vi "ATS_State_Device.vi"(6 "DevInfo_In":T3={"Handle"=0, "Board"="", "CPLD"="", "MemorySize"=0, "SampleSize"=0, "ID"=0, "High_Memory"=FALSE, "Chan/Board"=2}, 7 "Sys_In":T1={"MS_Mode"=FALSE, "MBoard"=0, "#Board"=1}, 8 "Ref_In":T2 {"Ranges (v)" format="%.2e"; "RangeB (v)" format="%.2e"; "RangeA (v)" format="%.2e"; "Clock (s)" format="%.2e"}, 9 "SetupIn":T5={"Record"={"Count"=1, "Presize"=512, "Length"=4096}, "Clock"={"ClckSource"=enum."Internal", "ClckRate"=16, "ClckEdge"=0, "Decimation"=0}, "Inputs"=[], "Trigger"={"TrigOperation"=enum."Only X", "Timeout (s)"=1.0, "Trig. Delay"=0, "Engine X"={"Source"=enum."Chan_A", "Slope"=enum."Positive", "Level"=128}, "Engine Y"={"Source"=enum."Disable", "Slope"=enum."Positive", "Level"=128}, "ExtTrigControl"={"Coupling"=enum."AC", "Range"=enum."1 V"}}} {"Inputs"."Range" items=["20mV", "40mV", "50mV", "80mV", "100mV", "200mV", "400mV", "500mV", "800mV", "1 V", "1.25 V", "2 V", "4 V", "5 V", "8 V", "10 V", "16 V", "20 V", "40 V", "HiFi"]; "Clock"."ClckEdge" items=["Rising", "Falling"]; "Clock"."ClckRate" items=["1 kS/s", "2 kS/s", "5 kS/s", "10 kS/s", "20 kS/s", "50 kS/s", "100 kS/s", "200 kS/s", "500 kS/s", "1 MS/s", "2 MS/s", "5 MS/s", "10 MS/s", "20 MS/s", "25 MS/s", "50 MS/s", "100 MS/s", "125 MS/s", "200 MS/s", "250 MS/s", "500 MS/s", "1 GS/s"]; "Trigger"."Timeout (s)" format="%.2f"}, 10 "DeviceIn":i32, 11 "ATS_GBL_Ctrl":T4=enum."Get") -> (0 "Ref_Out":T2 {"Ranges (v)" format="%.2e"; "RangeB (v)" format="%.2e"; "RangeA (v)" format="%.2e"; "Clock (s)" format="%.2e"}, 1 "SetupOut":T5={"Record"={"Count"=1, "Presize"=512, "Length"=4096}, "Clock"={"ClckSource"=enum."Internal", "ClckRate"=16, "ClckEdge"=0, "Decimation"=0}, "Inputs"=[], "Trigger"={"TrigOperation"=enum."Only X", "Timeout (s)"=1.0, "Trig. Delay"=0, "Engine X"={"Source"=enum."Chan_A", "Slope"=enum."Positive", "Level"=128}, "Engine Y"={"Source"=enum."Disable", "Slope"=enum."Positive", "Level"=128}, "ExtTrigControl"={"Coupling"=enum."AC", "Range"=enum."1 V"}}} {"Inputs"."Range" items=["20mV", "40mV", "50mV", "80mV", "100mV", "200mV", "400mV", "500mV", "800mV", "1 V", "1.25 V", "2 V", "4 V", "5 V", "8 V", "10 V", "16 V", "20 V", "40 V", "HiFi"]; "Clock"."ClckEdge" items=["Rising", "Falling"]; "Clock"."ClckRate" items=["1 kS/s", "2 kS/s", "5 kS/s", "10 kS/s", "20 kS/s", "50 kS/s", "100 kS/s", "200 kS/s", "500 kS/s", "1 MS/s", "2 MS/s", "5 MS/s", "10 MS/s", "20 MS/s", "25 MS/s", "50 MS/s", "100 MS/s", "125 MS/s", "200 MS/s", "250 MS/s", "500 MS/s", "1 GS/s"]; "Trigger"."Timeout (s)" format="%.2f"}, 2 "DeviceOut":i32, 3 "#Device":i32, 4 "DevInfo_Out":T3={"Handle"=0, "Board"="", "CPLD"="", "MemorySize"=0, "SampleSize"=0, "ID"=0, "High_Memory"=FALSE, "Chan/Board"=2}, 5 "Sys_Out":T1={"MS_Mode"=FALSE, "MBoard"=0, "#Board"=1})   [LabVIEW 2015]
doc: "_____AlazarTech, Scope_____\n\nState of all ATS device.\nDO NOT MODIFY."
uses:
  ATS_ctl/ATS_Global_4Ch.ctl
  ATS_ctl/Record.ctl
  ATS_ctl/Clock.ctl
  ATS_ctl/ClockSource.ctl
  ATS_ctl/ClockRate.ctl
  ATS_ctl/ClockEdge.ctl
  ATS_ctl/ATS_InputArray.ctl
  ATS_ctl/InputCtrl.ctl
  ATS_ctl/Coupling.ctl
  ATS_ctl/Range.ctl
  ATS_ctl/Impedance.ctl
  ATS_ctl/Bandwidth.ctl
  ATS_ctl/ATS_Trigger_4Ch.ctl
  ATS_ctl/TriggerOperation.ctl
  ATS_ctl/ATS_TriggerEngine_4Ch.ctl
  ATS_ctl/ATS_TriggerSource_4Ch.ctl
  ATS_ctl/ExtTrigger.ctl
  ATS_ctl/ExtTrigRange.ctl
  ATS_ctl/ATS_Global_Ctrl.ctl
  ATS_ctl/Device_Info.ctl
  ATS_ctl/ATS_Set_Value.ctl
  ATS_ctl/ATS_Sys_Info.ctl
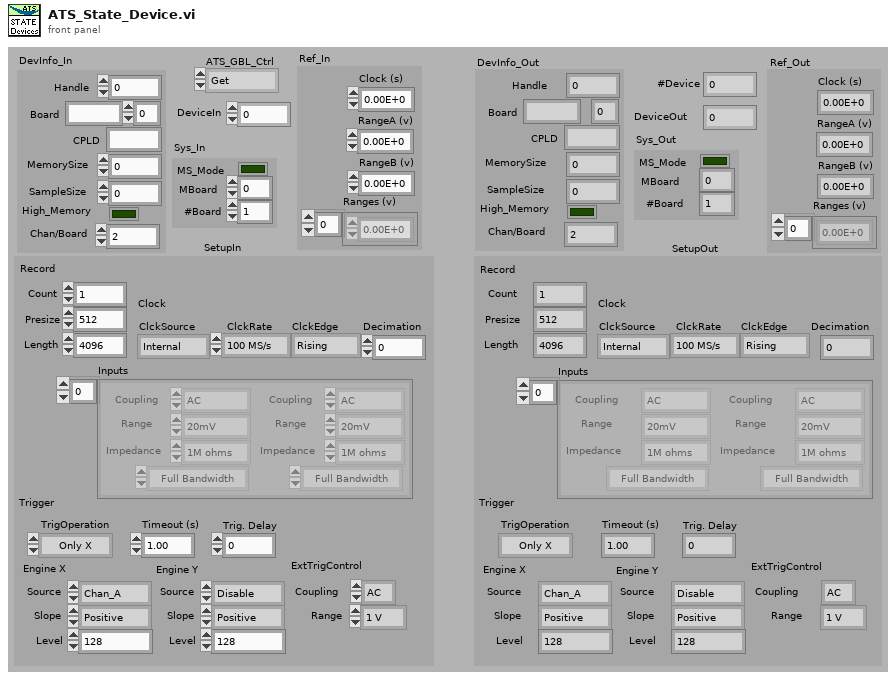
[diagram p1: front panel]
types:
  T1 = typedef "ATS_Sys_Info.ctl" = cluster{"MS_Mode":bool, "MBoard":i32, "#Board":i32}
  T2 = typedef "ATS_Set_Value.ctl" = cluster{"Clock (s)":dbl, "RangeA (v)":dbl, "RangeB (v)":dbl, "Ranges (v)":dbl[]}
  T3 = typedef "Device_Info.ctl" = cluster{"Handle":u32, "Board":string, "CPLD":string, "MemorySize":u32, "SampleSize":u8, "ID":i32, "High_Memory":bool, "Chan/Board":u8}
  T4 = typedef "ATS_Global_Ctrl.ctl" = enum16{"Init_Device", "Clear_ALL", "Set", "Get"}
  T5 = typedef "ATS_Global_4Ch.ctl" = cluster{"Record":T6, "Clock":T7, "Inputs":T11, "Trigger":T17}
  T6 = typedef "Record.ctl" = cluster{"Count":u32, "Presize":u32, "Length":u32}
  T7 = typedef "Clock.ctl" = cluster{"ClckSource":T8, "ClckRate":T9, "ClckEdge":T10, "Decimation":u32}
  T8 = typedef "ClockSource.ctl" = enum16{"Internal", "External", "Medium Ext.", "Slow Ext.", "Ext. AC", "Ext. DC", "Ext. (PLL)"}
  T9 = typedef "ClockRate.ctl" = u32
  T10 = typedef "ClockEdge.ctl" = u16
  T11 = typedef "ATS_InputArray.ctl" = T12[]
  T12 = typedef "InputCtrl.ctl" = cluster{"Coupling":T13, "Range":T14, "Impedance":T15, "Bandwidth":T16}
  T13 = typedef "Coupling.ctl" = enum16{"AC", "DC"}
  T14 = typedef "Range.ctl" = u32
  T15 = typedef "Impedance.ctl" = enum16{"1M ohms", "50 ohms"}
  T16 = typedef "Bandwidth.ctl" = enum16{"Full Bandwidth", "Reduce Bandwidth"}
  T17 = typedef "ATS_Trigger_4Ch.ctl" = cluster{"TrigOperation":T18, "Timeout (s)":dbl, "Trig. Delay":u32, "Engine X":T19, "Engine Y":T19, "ExtTrigControl":T21}
  T18 = typedef "TriggerOperation.ctl" = enum16{"Only X", "Only Y", "X or Y", "X and Y", "X xor Y", "X and not Y", "not X and Y"}
  T19 = typedef "ATS_TriggerEngine_4Ch.ctl" = cluster{"Source":T20, "Slope":enum32{"Positive", "Negative"}, "Level":u32}
  T20 = typedef "ATS_TriggerSource_4Ch.ctl" = enum32{"Chan_A", "Chan_B", "External", "Disable", "Chan_C", "Chan_D"}
  T21 = typedef "ExtTrigger.ctl" = cluster{"Coupling":T13, "Range":T22}
  T22 = typedef "ExtTrigRange.ctl" = enum16{"1 V", "5 V", "TTL"}
  T23 = cluster{"DevInfo_In":T3, "Ref_In":T2, "SetupIn":T5, "Sys_In":T1}
  T24 = cluster{"DevInfo_In":T3, "Ref_In":T2, "SetupIn":T5, "Sys_In":T1}[]
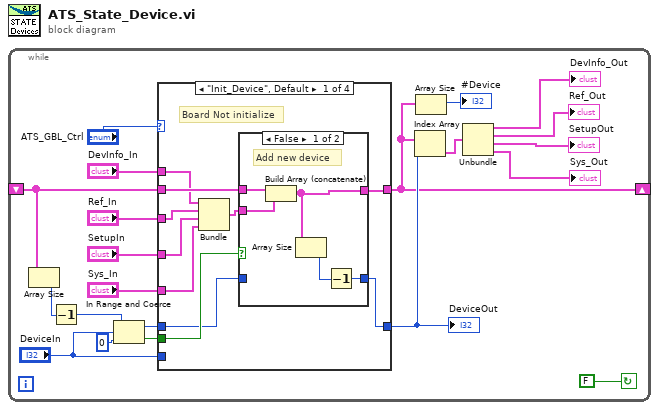
[diagram p0: block diagram]
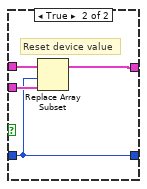
[diagram p2: hidden frame]
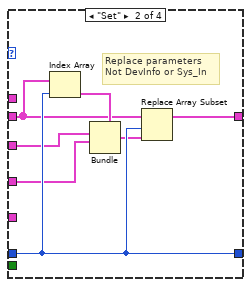
[diagram p3: hidden frame]
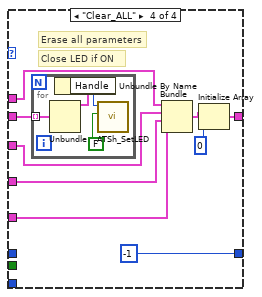
[diagram p5: hidden frame]
diagram:
  n1 = while {
    shift-right: [w7] -> _
    shift-left: _ -> [w8]
    stop <- FALSE continue-if-true
    n2 = Array Size(array=w8) -> (size(s)=w11:i32)
    n3 = Decrement(x=w11) -> (x-1=w10:i32)
    n4 = In Range and Coerce(upper limit=w10, x="DeviceIn", lower limit=0) -> (coerced(x)=w18:i32, In Range?=w12:bool)
    n5 = case shown="\"Init_Device\", Default" "ATS_GBL_Ctrl" {
      tunnel: w18 -> [w23 w47 w48 _]
      tunnel: "SetupIn" -> [w28 w42 _ w55]
      tunnel: [w22 w47 w48 -1 ("DeviceIn")] -> w13
      tunnel: "DeviceIn" -> [_ _ _ _]
      tunnel: "DevInfo_In" -> [w26 _ _ w54]
      tunnel: w12 -> [w31 _ _ _]
      tunnel: "Ref_In" -> [w27 w43 _ w56]
      tunnel: [w30 w44 w49 w52] -> w7
      tunnel: w8 -> [w29 w45 w49 w51]
      tunnel: "Sys_In" -> [w24 _ _ w50]
      frame "Init_Device", Default {
        # "Board Not initialize"
        n6 = Bundle("DevInfo_In"=w26, "Ref_In"=w27, "SetupIn"=w28, "Sys_In"=w24) -> (w25:T23)  [unwired: 1 in]
        n7 = case shown="False" w31 {
          tunnel: w23 -> [_ w37]
          tunnel: [w34 w39] -> w30
          tunnel: w29 -> [w36 w40]
          tunnel: w25 -> [w35 w38]
          tunnel: [w32 w37] -> w22
          frame False {
            # "Add new device"
            n8 = Build Array (concatenate)(w36, w35) -> (w34:T24)
            n9 = Array Size(array=w34) -> (size(s)=w33:i32)
            n10 = Decrement(x=w33) -> (x-1=w32:i32)
          }
          frame True {
            # "Reset device value"
            n11 = Replace Array Subset(array=w40, new element=w38, index=w37) -> (w39:T24)
          }
        }
      }
      frame "Set" {
        # "Replace parameters\nNot DevInfo or Sys_In"
        n12 = Index Array(array=w45, index=w47) -> (element=w46:T23)
        n13 = Bundle(cluster=w46, "Ref_In"=w43, "SetupIn"=w42) -> (w41:T23)  [unwired: 2 in]
        n14 = Replace Array Subset(array=w45, new element=w41, index=w47) -> (w44:T24)
      }
      frame "Get" {
        # "Read parameters"
      }
      frame "Clear_ALL" {
        # "Close LED if ON"
        # "Erase all parameters"
        n15 = for {
          tunnel: w51 -> [w62] mode=indexing
          n16 = Unbundle(w62) -> ("DevInfo_In"=w61:T3)  [unwired: 3 out]
          n17 = Unbundle By Name(w61) -> ("Handle"=w60:u32)
          n18 = call "ATSh_SetLED.vi"("state"=FALSE, "Handle"=w60) -> ()  [unwired: 5 in, 1 out]
        }
        n19 = Bundle("DevInfo_In"=w54, "Ref_In"=w56, "SetupIn"=w55, "Sys_In"=w50) -> (w53:T23)  [unwired: 1 in]
        n20 = Initialize Array(w53, 0 ("dimension size")) -> (w52:T24)
      }
    }
    "DeviceOut" <- w13
    n21 = Index Array(array=w7, index=w13) -> (element=w6:T23)
    n22 = Array Size(array=w7) -> (size(s)=→"#Device":i32)
    n23 = Unbundle(w6) -> ("DevInfo_In"=→"DevInfo_Out":T3, "Ref_In"=→"Ref_Out":T2, "SetupIn"=→"SetupOut":T5, "Sys_In"=→"Sys_Out":T1)
  }
